vi "CYCLE_PLAN_CREATOR_COUNT_LOGIC.vi"(7 "FG CAT No":string, 8 "error in (no error)":errorcluster, 9 "BLOCK NO":string, 10 "Qty":u16=1 min=1 max=90 step=1, 11 "all rows IN":string[][](array[string])) -> (0 "error out":errorcluster, 3 "all rows OUT":string[][](array[string]))   [LabVIEW 2017]
uses:
  <vilib>/Utility/file.llb/Read Delimited Spreadsheet (string).vi
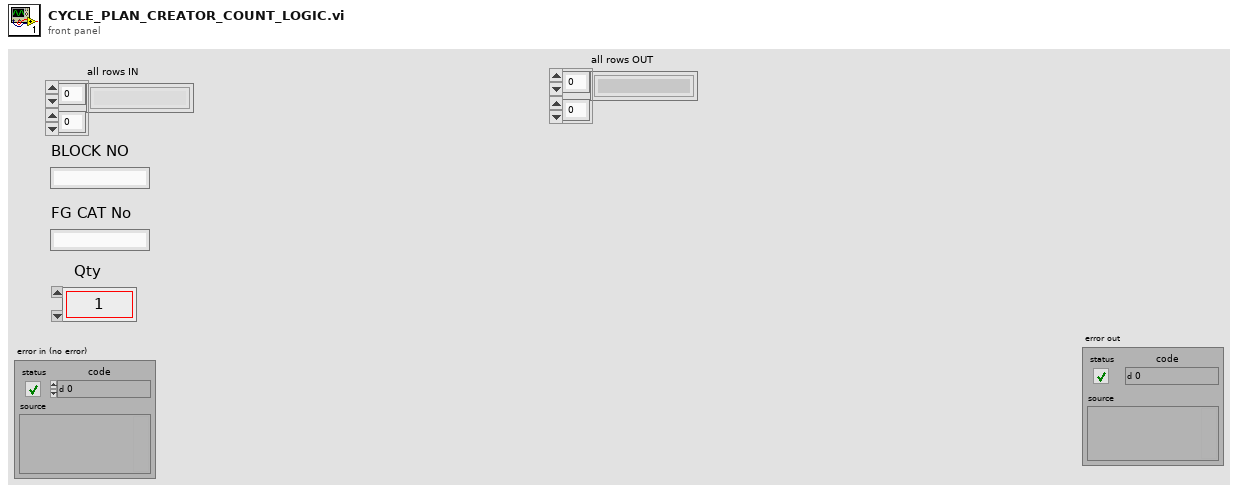
[diagram p1: front panel]
types:
  T1 = enum32{"invalid app kind", "Development System", "Run Time System", "Student Edition", "Embedded LabVIEW", "Evaluation", "Custom"}
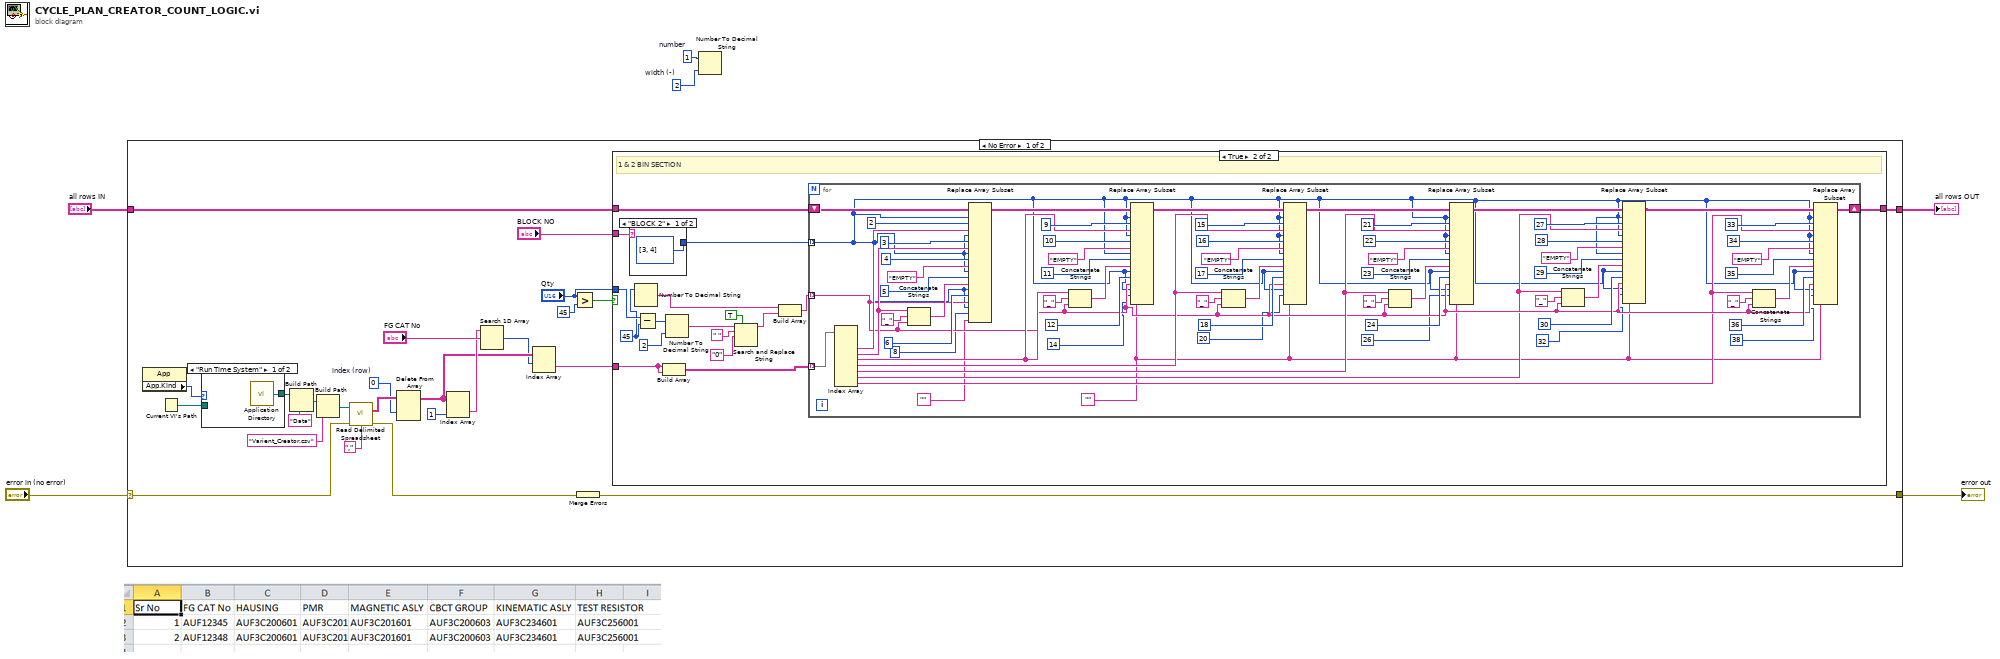
[diagram p0: block diagram]
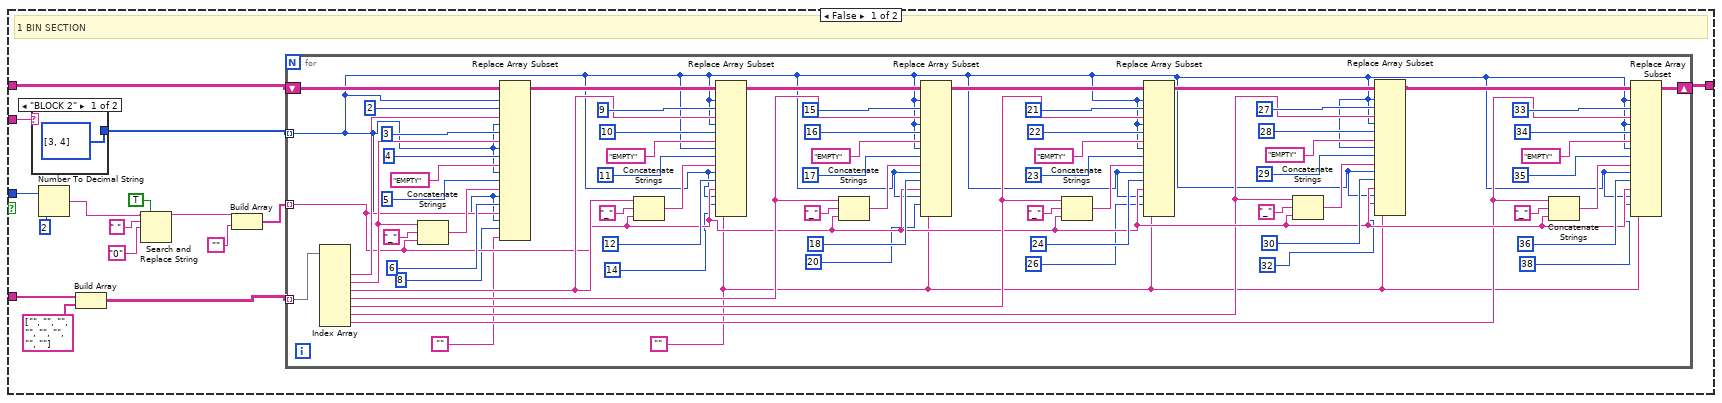
[diagram p2: hidden frame]
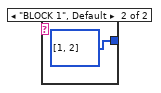
[diagram p3: hidden frame]
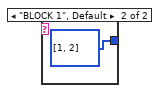
[diagram p4: hidden frame]
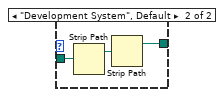
[diagram p5: hidden frame]
diagram:
  w1 = i16 2  # width (-)
  w2 = 1  # number
  n1 = case shown="No Error" "error in (no error)" {
    selector: "error in (no error)" -> [w22 w210]
    tunnel: [w31 w210] -> w5
    tunnel: [w8 w209] -> w4
    tunnel: "all rows IN" -> [w10 w209]
    frame No Error {
      w19 = 0  # index (row)
      n2 = property class="App"() -> ("App.Kind"=w29:T1)  [unwired: 2 in, 2 out]
      n3 = Current VI's Path() -> (path=w30:path)
      n4 = case shown="\"Run Time System\"" w29 {
        tunnel: w30 -> [_ w207]
        tunnel: [w205 w206] -> w26
        frame "Run Time System" {
          n5 = call <vilib>:"Application Directory.vi"() -> ("Application Directory"=w205:path)
        }
        frame "Development System", Default {
          n6 = Strip Path(path=w207) -> (stripped path=w208:path)  [unwired: 1 out]
          n7 = Strip Path(path=w208) -> (stripped path=w206:path)  [unwired: 1 out]
        }
      }
      n8 = Build Path(base path=w26, name or relative path="Data") -> (appended path=w27:path)
      n9 = Build Path(base path=w27, name or relative path="Varient_Creator.csv") -> (appended path=w24:path)
      n10 = call-poly <vilib>:"Read Delimited Spreadsheet.vi"("file path (dialog if empty)"=w24, "error in (no error)"=w22, "delimiter (\\t)"=",") -> ("all rows"=w20:string[][], "error out"=w21:errorcluster)  [unwired: 7 in, 4 out]
      n11 = Delete From Array(array=w20, index (row)=w19) -> (array with subset deleted=w15:string[][])  [unwired: 2 in, 1 out]
      n12 = Index Array(array=w15, index (col)=1) -> (element=w16:string[])  [unwired: 1 in]
      n13 = Search 1D Array(1D array=w16, element="FG CAT No") -> (index of element=w14:i32)  [unwired: 1 in]
      n14 = Index Array(array=w15, index (row)=w14) -> (element=w9:string[])  [unwired: 1 in]
      n15 = Greater?(x="Qty", y=u16 45) -> (0:w12:bool)
      n16 = Merge Errors(w21) -> (w31:errorcluster)
      n17 = case shown="True" w12 {
        tunnel: "BLOCK NO" -> [w46 w133]
        tunnel: w10 -> [w42 w131]
        tunnel: w9 -> [w44 w127]
        tunnel: [w38 w134] -> w8
        tunnel: "Qty" -> [w47 w126]
        frame False {
          # "1 BIN SECTION"
          n18 = case shown="\"BLOCK 2\"" w46 {
            tunnel: [i32[] [3, 4] i32[] [1, 2]] -> w41
            frame "BLOCK 2" {
            }
            frame "BLOCK 1", Default {
            }
          }
          n19 = Number To Decimal String(number=w47, width (-)=u16 2) -> (decimal integer string=w33:string)
          n20 = Build Array(w44, string[] ["", "", "", "", "", "", "", ""]) -> (w39:string[][])
          n21 = Search and Replace String(replace all?=TRUE, input string=w33, search string=" ", replace string="0") -> (result string=w32:string)  [unwired: 4 in, 3 out]
          n22 = Build Array(w32, "") -> (w40:string[])
          n23 = for {
            tunnel: w39 -> [w115] mode=indexing
            tunnel: w40 -> [w60] mode=indexing
            tunnel: w41 -> [w50] mode=indexing
            shift-right: [w61] -> w38
            shift-left: w42 -> [w57]
            w48 = ""
            n24 = Index Array(array=w115) -> (element #2=w113:string, element #3=w108:string, element #4=w96:string, element #5=w87:string, element #6=w78:string, element #7=w59:string, element #8=w58:string)  [unwired: 8 in, 1 out]
            n25 = Concatenate Strings(w108, "_", w60) -> (w106:string)
            n26 = Replace Array Subset(array=w57, new element #1=w113, index (row) #1=w50, index (col) #1=u16 2, new element #2=w108, index (row) #2=w50, index (col) #2=u16 3, new element #3="EMPTY", index (row) #3=w50, index (col) #3=u16 4, new element #4=w106, index (row) #4=w50, index (col) #4=u16 5, new element #5=w60, index (row) #5=w50, index (col) #5=u16 6, new element #6="", index (row) #6=w50, index (col) #6=u16 8) -> (w97:string[][])
            n27 = Concatenate Strings(w96, "_", w60) -> (w103:string)
            n28 = Replace Array Subset(array=w97, new element #1=w96, index (row) #1=w50, index (col) #1=u16 9, new element #2="EMPTY", index (row) #2=w50, index (col) #2=u16 10, new element #3=w103, index (row) #3=w50, index (col) #3=u16 11, new element #4=w60, index (row) #4=w50, index (col) #4=u16 12, new element #5=w48, index (row) #5=w50, index (col) #5=u16 14) -> (w88:string[][])
            n29 = Concatenate Strings(w87, "_", w60) -> (w90:string)
            n30 = Replace Array Subset(array=w88, new element #1=w87, index (row) #1=w50, index (col) #1=u16 15, new element #2="EMPTY", index (row) #2=w50, index (col) #2=u16 16, new element #3=w90, index (row) #3=w50, index (col) #3=u16 17, new element #4=w60, index (row) #4=w50, index (col) #4=u16 18, new element #5=w48, index (row) #5=w50, index (col) #5=u16 20) -> (w79:string[][])
            n31 = Concatenate Strings(w78, "_", w60) -> (w85:string)
            n32 = Replace Array Subset(array=w79, new element #1=w78, index (row) #1=w50, index (col) #1=u16 21, new element #2="EMPTY", index (row) #2=w50, index (col) #2=u16 22, new element #3=w85, index (row) #3=w50, index (col) #3=u16 23, new element #4=w60, index (row) #4=w50, index (col) #4=u16 24, new element #5=w48, index (row) #5=w50, index (col) #5=u16 26) -> (w63:string[][])
            n33 = Concatenate Strings(w59, "_", w60) -> (w72:string)
            n34 = Replace Array Subset(array=w63, new element #1=w59, index (row) #1=w50, index (col) #1=u16 27, new element #2="EMPTY", index (row) #2=w50, index (col) #2=u16 28, new element #3=w72, index (row) #3=w50, index (col) #3=u16 29, new element #4=w60, index (row) #4=w50, index (col) #4=u16 30, new element #5=w48, index (row) #5=w50, index (col) #5=u16 32) -> (w62:string[][])
            n35 = Concatenate Strings(w58, "_", w60) -> (w69:string)
            n36 = Replace Array Subset(array=w62, new element #1=w58, index (row) #1=w50, index (col) #1=u16 33, new element #2="EMPTY", index (row) #2=w50, index (col) #2=u16 34, new element #3=w69, index (row) #3=w50, index (col) #3=u16 35, new element #4=w60, index (row) #4=w50, index (col) #4=u16 36, new element #5=w48, index (row) #5=w50, index (col) #5=u16 38) -> (w61:string[][])
          }
        }
        frame True {
          w124 = u16 45
          # "1 & 2 BIN SECTION"
          n37 = case shown="\"BLOCK 2\"" w133 {
            tunnel: [i32[] [3, 4] i32[] [1, 2]] -> w132
            frame "BLOCK 2" {
            }
            frame "BLOCK 1", Default {
            }
          }
          n38 = Number To Decimal String(number=w124) -> (decimal integer string=w128:string)  [unwired: 1 in]
          n39 = Subtract(x=w126, y=w124) -> (x-y=w125:u16)
          n40 = Build Array(w127, w127) -> (w129:string[][])
          n41 = Number To Decimal String(number=w125, width (-)=u16 2) -> (decimal integer string=w119:string)
          n42 = Search and Replace String(replace all?=TRUE, input string=w119, search string=" ", replace string="0") -> (result string=w121:string)  [unwired: 4 in, 3 out]
          n43 = Build Array(w128, w121) -> (w130:string[])
          n44 = for {
            tunnel: w129 -> [w202] mode=indexing
            tunnel: w130 -> [w147] mode=indexing
            tunnel: w132 -> [w137] mode=indexing
            shift-right: [w148] -> w134
            shift-left: w131 -> [w144]
            w135 = ""
            n45 = Index Array(array=w202) -> (element #2=w200:string, element #3=w195:string, element #4=w183:string, element #5=w174:string, element #6=w165:string, element #7=w146:string, element #8=w145:string)  [unwired: 8 in, 1 out]
            n46 = Concatenate Strings(w195, "_", w147) -> (w193:string)
            n47 = Replace Array Subset(array=w144, new element #1=w200, index (row) #1=w137, index (col) #1=u16 2, new element #2=w195, index (row) #2=w137, index (col) #2=u16 3, new element #3="EMPTY", index (row) #3=w137, index (col) #3=u16 4, new element #4=w193, index (row) #4=w137, index (col) #4=u16 5, new element #5=w147, index (row) #5=w137, index (col) #5=u16 6, new element #6="", index (row) #6=w137, index (col) #6=u16 8) -> (w184:string[][])
            n48 = Concatenate Strings(w183, "_", w147) -> (w190:string)
            n49 = Replace Array Subset(array=w184, new element #1=w183, index (row) #1=w137, index (col) #1=u16 9, new element #2="EMPTY", index (row) #2=w137, index (col) #2=u16 10, new element #3=w190, index (row) #3=w137, index (col) #3=u16 11, new element #4=w147, index (row) #4=w137, index (col) #4=u16 12, new element #5=w135, index (row) #5=w137, index (col) #5=u16 14) -> (w175:string[][])
            n50 = Concatenate Strings(w174, "_", w147) -> (w177:string)
            n51 = Replace Array Subset(array=w175, new element #1=w174, index (row) #1=w137, index (col) #1=u16 15, new element #2="EMPTY", index (row) #2=w137, index (col) #2=u16 16, new element #3=w177, index (row) #3=w137, index (col) #3=u16 17, new element #4=w147, index (row) #4=w137, index (col) #4=u16 18, new element #5=w135, index (row) #5=w137, index (col) #5=u16 20) -> (w166:string[][])
            n52 = Concatenate Strings(w165, "_", w147) -> (w172:string)
            n53 = Replace Array Subset(array=w166, new element #1=w165, index (row) #1=w137, index (col) #1=u16 21, new element #2="EMPTY", index (row) #2=w137, index (col) #2=u16 22, new element #3=w172, index (row) #3=w137, index (col) #3=u16 23, new element #4=w147, index (row) #4=w137, index (col) #4=u16 24, new element #5=w135, index (row) #5=w137, index (col) #5=u16 26) -> (w150:string[][])
            n54 = Concatenate Strings(w146, "_", w147) -> (w159:string)
            n55 = Replace Array Subset(array=w150, new element #1=w146, index (row) #1=w137, index (col) #1=u16 27, new element #2="EMPTY", index (row) #2=w137, index (col) #2=u16 28, new element #3=w159, index (row) #3=w137, index (col) #3=u16 29, new element #4=w147, index (row) #4=w137, index (col) #4=u16 30, new element #5=w135, index (row) #5=w137, index (col) #5=u16 32) -> (w149:string[][])
            n56 = Concatenate Strings(w145, "_", w147) -> (w156:string)
            n57 = Replace Array Subset(array=w149, new element #1=w145, index (row) #1=w137, index (col) #1=u16 33, new element #2="EMPTY", index (row) #2=w137, index (col) #2=u16 34, new element #3=w156, index (row) #3=w137, index (col) #3=u16 35, new element #4=w147, index (row) #4=w137, index (col) #4=u16 36, new element #5=w135, index (row) #5=w137, index (col) #5=u16 38) -> (w148:string[][])
          }
        }
      }
    }
    frame Error {
    }
  }
  "error out" <- w5
  "all rows OUT" <- w4
  n58 = Number To Decimal String(number=w2, width (-)=w1) -> ()  [unwired: 1 out]
